vi "SetTrigger.vi"(8 "error in (no error)":errorcluster, 10 "Trigger":T1, 11 "ScopeBase In":refnum<class "ScopeBase.lvclass">) -> (0 "error out":errorcluster, 3 "ScopeBase Out":refnum<class "ScopeBase.lvclass">)   [LabVIEW 2013, in "ScopeBase.lvclass"]
uses:
  ScopeBase.lvclass
  Scope5782/Scope/controls/5782_trigger_type.ctl
  ScopeBase.lvclass/ScopeBase.ctl
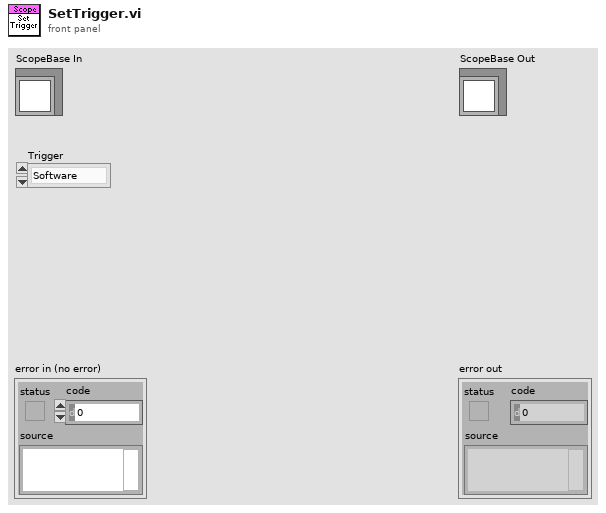
[diagram p1: front panel]
types:
  T1 = typedef "5782_trigger_type.ctl" = enum16{"Software", "Trigger input"}
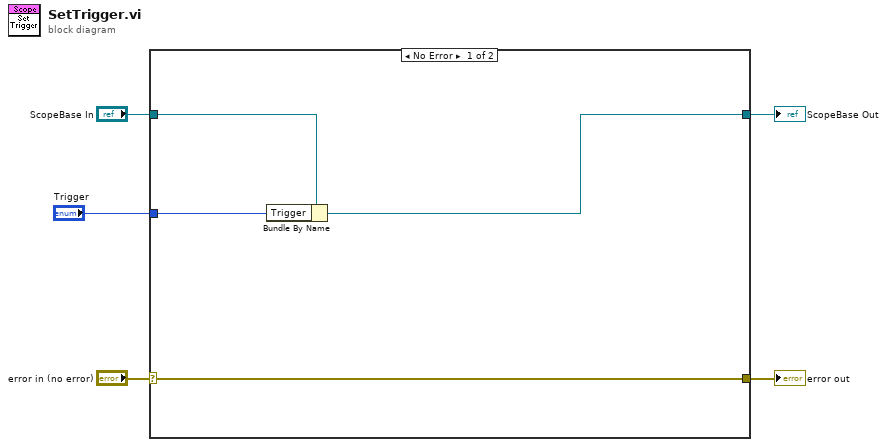
[diagram p0: block diagram]
diagram:
  n1 = case shown="No Error" "error in (no error)" {
    selector: "error in (no error)" -> [w9 w11]
    tunnel: [w9 w11] -> w3
    tunnel: [w6 w10] -> w4
    tunnel: "ScopeBase In" -> [w7 w10]
    tunnel: "Trigger" -> [w8 _]
    frame No Error {
      n2 = Bundle By Name(cluster=w7, "Trigger"=w8) -> (w6:refnum<class "ScopeBase.lvclass">)
    }
    frame Error {
    }
  }
  "error out" <- w3
  "ScopeBase Out" <- w4
